vi "Update Value.vi"(6 "Time":dbl, 8 "error in (no error)":errorcluster, 11 "HtmlButtonControl in":refnum<class "HttpButtonControl.lvclass">) -> (0 "error out":errorcluster, 1 "Update":bool, 2 "Value":variant, 3 "HtmlButtonControl out":refnum<class "HttpButtonControl.lvclass">)   [LabVIEW 2020, in "VolatusGUIElements.lvlib" / "HttpButtonControl.lvclass"]
uses:
  HttpButtonControl.lvclass
  HttpButtonControl.lvclass/HttpButtonControl.ctl
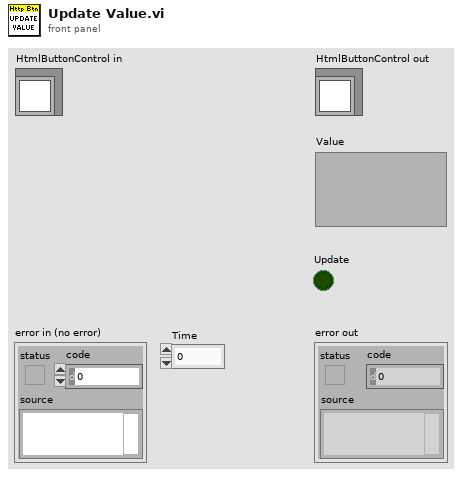
[diagram p1: front panel]
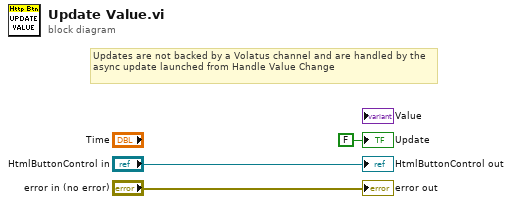
[diagram p0: block diagram]
diagram:
  # "Updates are not backed by a Volatus channel and are handled by the async update launched from Handle Value Change"
  "error out" <- "error in (no error)"
  "HtmlButtonControl out" <- "HtmlButtonControl in"
  "Update" <- FALSE ("Update")
